vi "svx_Continuous Multitone Waveform.vi"(6 "sampling info":cluster{"Fs":dbl, "#s":dbl}={"Fs"=1000.0, "#s"=1000.0} {"Fs" format="%.2p"}, 7 "generation control":T2(ring), 8 "error in":errorcluster, 9 "delay until transition (0 samples)":i32, 10 "initial waveform state":T1 {"relative amplitudes" format="%.2p"; "frequencies" format="%.2p"; "tf" format="%.2f"; "offset" format="%.2f"; "phases" format="%.2f"; "total amplitude" format="%.2f"}, 11 "desired waveform state":T3={"frequencies"=[], "relative amplitudes"=[], "phases"=[], "total amplitude"=1.0, "offset"=0.0, "tf (ignored)"=0.0} {"relative amplitudes" format="%.2p"; "frequencies" format="%.2p"; "tf (ignored)" format="%.2f"; "phases" format="%.2f"; "offset" format="%.2p"; "total amplitude" format="%.2p"}) -> (0 "error out":errorcluster, 1 "index of transition":i32, 2 "final waveform state":T1 {"relative amplitudes" format="%.2p"; "frequencies" format="%.2p"; "tf" format="%.2f"; "offset" format="%.2f"; "phases" format="%.2f"; "total amplitude" format="%.2f"}, 3 "signal out":waveform(dbl))   [LabVIEW 2017]
uses:
  <vilib>/Analysis/NI_AALBase.lvlib
panel:
  # "You cannot change the number of tones\nand maintain continuity"
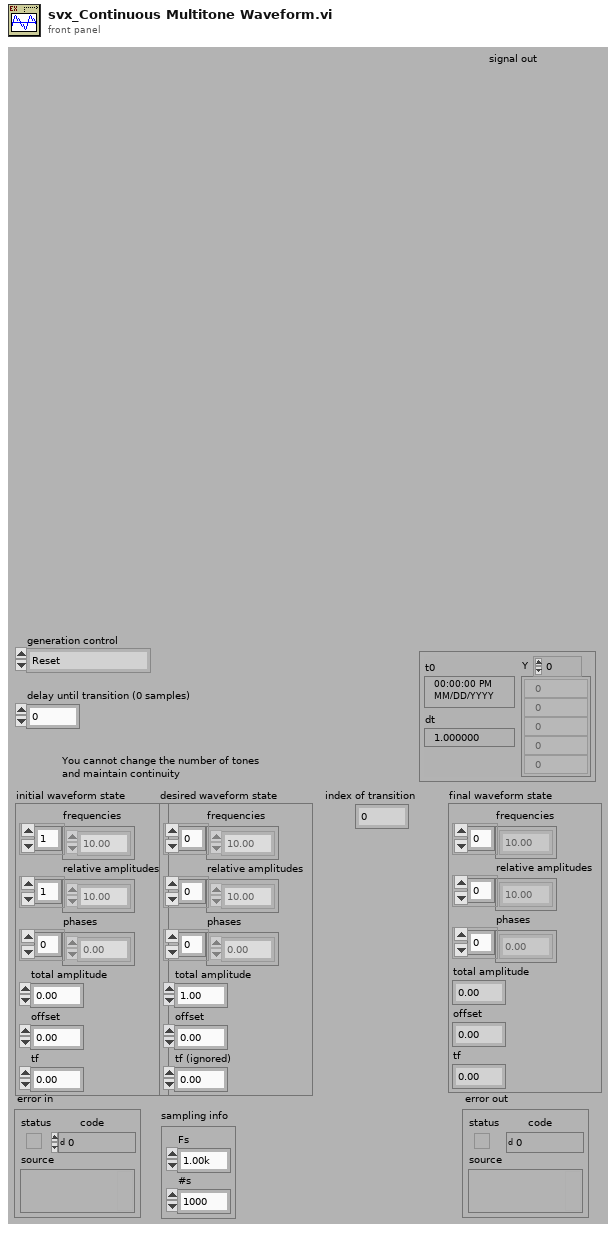
[diagram p1: front panel]
types:
  T1 = cluster{"frequencies":dbl[], "relative amplitudes":dbl[], "phases":dbl[], "total amplitude":dbl, "offset":dbl, "tf":dbl}
  T2 = enum16{"Reset", "Continue from previous", "Continue from state", "Zero from previous", "Zero from state"}
  T3 = cluster{"frequencies":dbl[], "relative amplitudes":dbl[], "phases":dbl[], "total amplitude":dbl, "offset":dbl, "tf (ignored)":dbl}
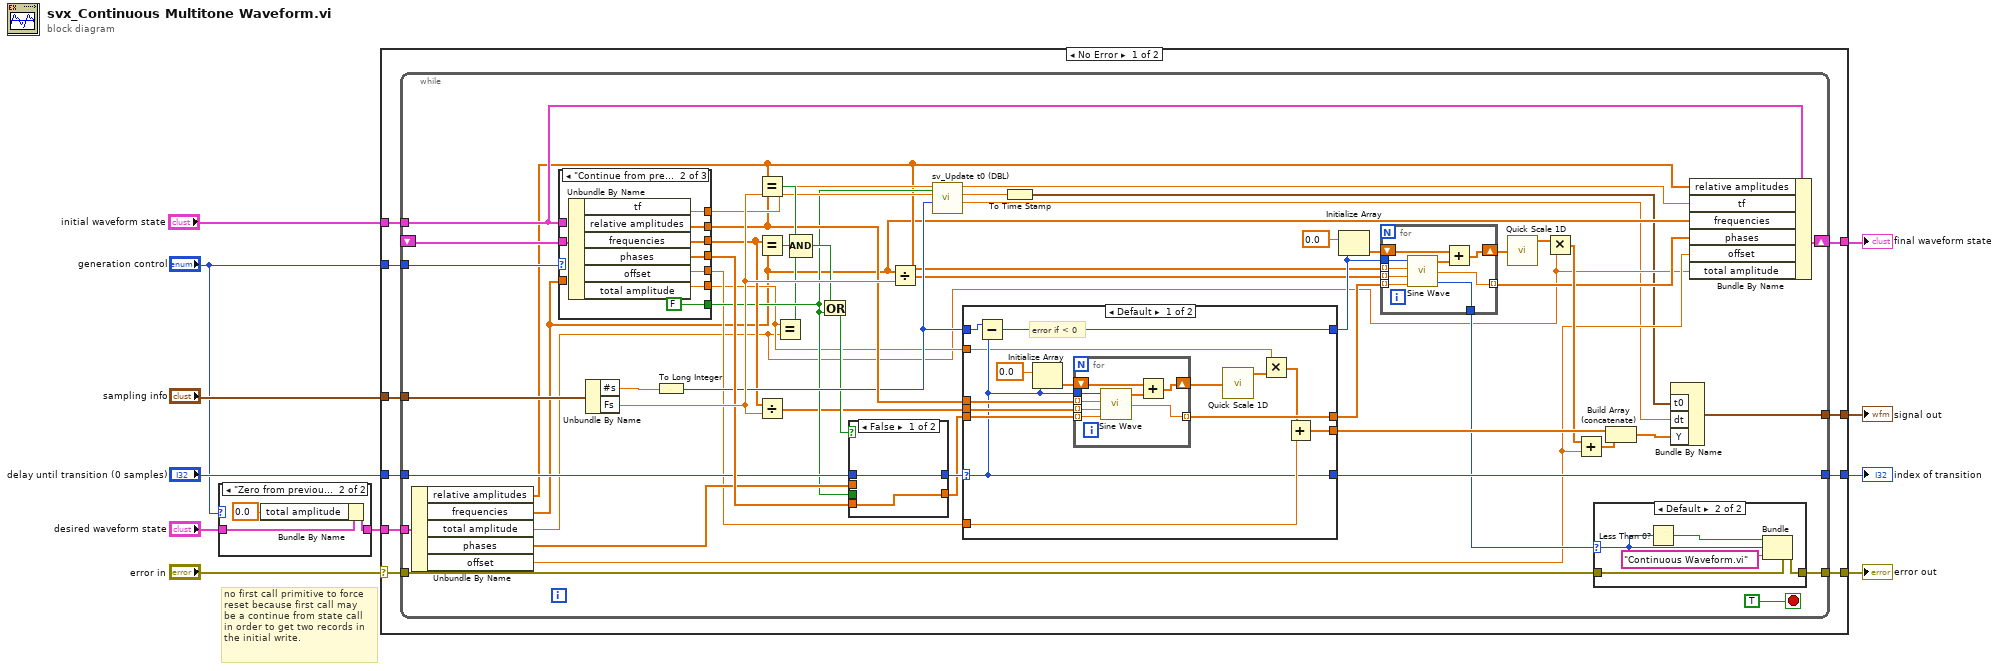
[diagram p0: block diagram]
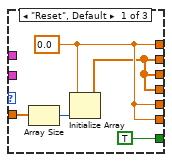
[diagram p4: hidden frame]
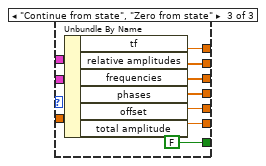
[diagram p5: hidden frame]
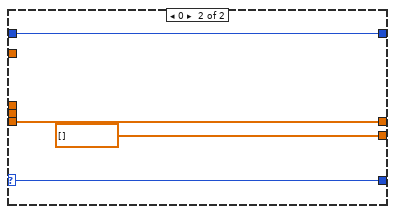
[diagram p6: hidden frame]
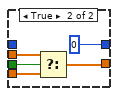
[diagram p7: hidden frame]
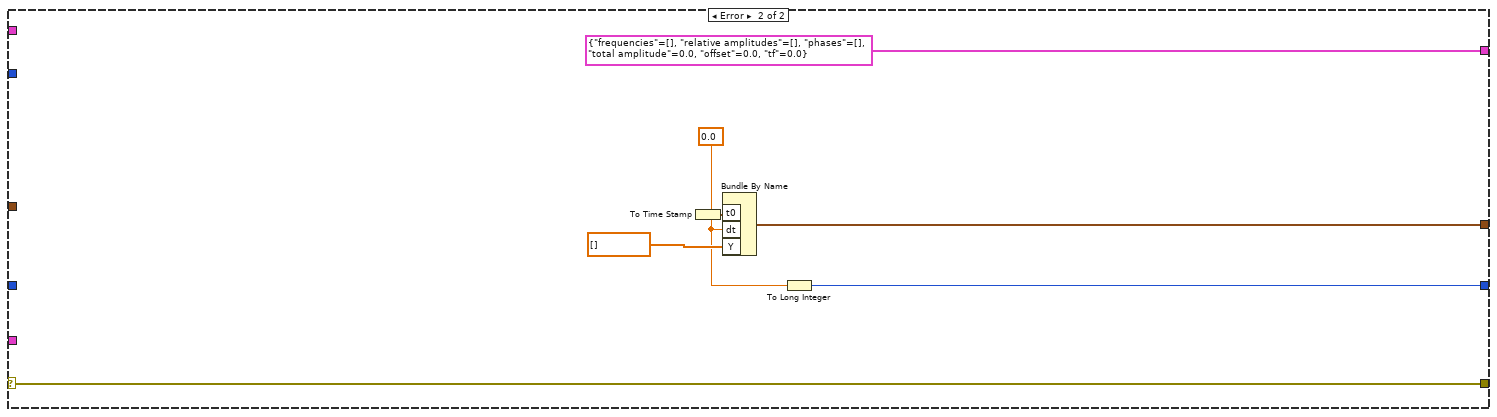
[diagram p8: hidden frame]
diagram:
  # "no first call primitive to force \nreset because first call may \nbe a continue from state call\nin order to get two records in \nthe initial write."
  n1 = case shown="\"Zero from previous\", \"Zero from state\"" "generation control" {
    tunnel: "desired waveform state" -> [w12 w14]
    tunnel: [w12 w13] -> w3
    frame Default {
    }
    frame "Zero from previous", "Zero from state" {
      n2 = Bundle By Name(cluster=w14, "total amplitude"=0.0) -> (w13:T3)
    }
  }
  n3 = case shown="No Error" "error in" {
    selector: "error in" -> [w22 w153]
    tunnel: "sampling info" -> [w25 _]
    tunnel: [w24 w153] -> w10
    tunnel: [w23 w154] -> w2
    tunnel: [w21 w150] -> w9
    tunnel: "delay until transition (0 samples)" -> [w20 _]
    tunnel: [w19 T1 {"frequencies"=[], "relative amplitudes"=[], "phases"=[], "total amplitude"=0.0, "offset"=0.0, "tf"=0.0} ("initial waveform state")] -> w7
    tunnel: "generation control" -> [w18 _]
    tunnel: w3 -> [w17 _]
    tunnel: "initial waveform state" -> [w16 _]
    frame No Error {
      n4 = while {
        tunnel: w16 -> [w52]
        tunnel: w17 -> [w60]
        tunnel: w18 -> [w67]
        shift-left: _ -> [w66]
        shift-right: [w32] -> w19
        tunnel: w20 -> [w57]
        tunnel: [w73] -> w21
        tunnel: w22 -> [w50]
        tunnel: [w75] -> w23
        tunnel: [w49] -> w24
        tunnel: w25 -> [w76]
        stop <- TRUE stop-if-true
        n5 = Unbundle By Name(w60) -> ("relative amplitudes"=w30:dbl[], "frequencies"=w29:dbl[], "total amplitude"=w28:dbl, "phases"=w59:dbl[], "offset"=w31:dbl)
        n6 = case shown="\"Continue from previous\", \"Zero from previous\"" w67 {
          tunnel: w66 -> [_ w104 _]
          tunnel: [TRUE FALSE FALSE] -> w54
          tunnel: [w94 w99 w108] -> w65
          tunnel: [w93 w103 w110] -> w64
          tunnel: [w93 w102 w112] -> w56
          tunnel: [w93 w101 w109] -> w63
          tunnel: [w94 w100 w111] -> w51
          tunnel: w52 -> [_ _ w107]
          tunnel: w29 -> [w95 _ _]
          tunnel: [w94 w98 w106] -> w38
          frame "Reset", Default {
            w94 = 0.0
            n7 = Array Size(array=w95) -> (size(s)=w96:i32)
            n8 = Initialize Array(w94, w96) -> (w93:dbl[])
          }
          frame "Continue from previous", "Zero from previous" {
            n9 = Unbundle By Name(w104) -> ("tf"=w99:dbl, "relative amplitudes"=w103:dbl[], "frequencies"=w102:dbl[], "phases"=w101:dbl[], "offset"=w100:dbl, "total amplitude"=w98:dbl)
          }
          frame "Continue from state", "Zero from state" {
            n10 = Unbundle By Name(w107) -> ("tf"=w108:dbl, "relative amplitudes"=w110:dbl[], "frequencies"=w112:dbl[], "phases"=w109:dbl[], "offset"=w111:dbl, "total amplitude"=w106:dbl)
          }
        }
        n11 = Unbundle By Name(w76) -> ("#s"=w58:dbl, "Fs"=w71:dbl)
        n12 = To Long Integer(number=w58) -> (32bit integer=w61:i32)
        n13 = Equal?(x=w30, y=w64) -> (x = y?=w74:bool)
        n14 = Equal?(x=w56, y=w29) -> (x = y?=w41:bool)
        n15 = Divide(x=w56, y=w71) -> (x/y=w48:dbl[])
        n16 = Equal?(x=w38, y=w28) -> (x = y?=w40:bool)
        n17 = Compound Arithmetic op=AND(w74, w41, w40) -> (w55:bool)
        n18 = Or(x=w55, y=w54) -> (x .or. y?=w53:bool)
        n19 = case shown="False" w53 {
          tunnel: [w142 w143] -> w34
          tunnel: w63 -> [w142 w144]
          tunnel: w57 -> [w141 _]
          tunnel: w59 -> [_ w145]
          tunnel: [w141 0] -> w47
          tunnel: w54 -> [_ w146]
          frame False {
          }
          frame True {
            n20 = Select(t=w145, s=w146, f=w144) -> (s? t:f=w143:dbl[])
          }
        }
        n21 = Divide(x=w29, y=w71) -> (x/y=w43:dbl[])
        n22 = call <vilib>:"sv_Update t0 (DBL).vi"("Reset Generation"=w54, "samples"=w61, "sample rate (S/s)"=w71, "tf previous"=w65) -> ("dt"=w26:dbl, "t0"=w62:dbl, "tf new"=w68:dbl)  [unwired: 5 in]
        n23 = case shown="Default" w47 {
          selector: w47 -> [w118 w137]
          tunnel: [w124 w138] -> w39
          tunnel: w61 -> [w125 w139]
          tunnel: w64 -> [w128 _]
          tunnel: [w118 w137] -> w73
          tunnel: [w126 dbl[] [] ("Sine Wave")] -> w72
          tunnel: [w127 w139] -> w46
          tunnel: w48 -> [w122 _]
          tunnel: w51 -> [w123 _]
          tunnel: w34 -> [w121 w138]
          tunnel: w38 -> [w115 _]
          frame Default {
            # "error if < 0"
            n24 = Subtract(x=w125, y=w118) -> (x-y=w127:i32)
            n25 = Initialize Array(0.0 ("element"), w118) -> (w119:dbl[])
            n26 = for {
              tunnel: w128 -> [w136] mode=indexing
              tunnel: w122 -> [w135] mode=indexing
              tunnel: w121 -> [w134] mode=indexing
              tunnel: w118 -> [w133]
              tunnel: [w132] -> w124 mode=indexing
              shift-right: [w129] -> w117
              shift-left: w119 -> [w131]
              n27 = call <vilib>:"Sine Wave.vi"("samples"=w133, "amplitude"=w136, "frequency"=w135, "phase in"=w134) -> ("sine wave"=w130:dbl[], "phase out"=w132:dbl)  [unwired: 1 in, 1 out]
              n28 = Add(x=w131, y=w130) -> (x+y=w129:dbl[])
            }
            n29 = call <vilib>:"Quick Scale 1D.vi"("X"=w117) -> ("Y[i]=X[i]/Max|X|"=w116:dbl[])  [unwired: 2 out]
            n30 = Multiply(x=w115, y=w116) -> (x*y=w114:dbl[])
            n31 = Add(x=w114, y=w123) -> (x+y=w126:dbl[])
          }
          frame 0 {
          }
        }
        n32 = To Time Stamp(1:w62) -> (0:w27:timestamp)
        n33 = Initialize Array(0.0 ("element"), w46) -> (w45:dbl[])
        n34 = for {
          tunnel: w30 -> [w86] mode=indexing
          tunnel: w43 -> [w85] mode=indexing
          tunnel: w39 -> [w84] mode=indexing
          tunnel: w46 -> [w83]
          tunnel: [w82] -> w33 mode=indexing
          shift-right: [w79] -> w37
          shift-left: w45 -> [w81]
          tunnel: [w78] -> w42
          n35 = call <vilib>:"Sine Wave.vi"("samples"=w83, "amplitude"=w86, "frequency"=w85, "phase in"=w84) -> ("sine wave"=w80:dbl[], "phase out"=w82:dbl, "error"=w78:i32)  [unwired: 1 in]
          n36 = Add(x=w81, y=w80) -> (x+y=w79:dbl[])
        }
        n37 = call <vilib>:"Quick Scale 1D.vi"("X"=w37) -> ("Y[i]=X[i]/Max|X|"=w35:dbl[])  [unwired: 2 out]
        n38 = Multiply(x=w35, y=w28) -> (x*y=w36:dbl[])
        n39 = Add(x=w36, y=w31) -> (x+y=w70:dbl[])
        n40 = case shown="Default" w42 {
          selector: w42 -> [_ w91]
          tunnel: w50 -> [w87 w92]
          tunnel: [w87 w88] -> w49
          frame 0 {
          }
          frame Default {
            n41 = Less Than 0?(x=w91) -> (x < 0?=w90:bool)
            n42 = Bundle(cluster=w92, "status"=w90, "code"=w91, "source"="Continuous Waveform.vi" ("subVI Name")) -> (w88:errorcluster)
          }
        }
        n43 = Build Array (concatenate)(w72, w70) -> (w69:dbl[])
        n44 = Bundle By Name("t0"=w27, "dt"=w26, "Y"=w69) -> (w75:waveform(dbl))  [unwired: 1 in]
        n45 = Bundle By Name(cluster=w52, "relative amplitudes"=w30, "tf"=w68, "frequencies"=w29, "phases"=w33, "offset"=w31, "total amplitude"=w28) -> (w32:T1)
      }
    }
    frame Error {
      w151 = 0.0 ("t0")
      n46 = To Time Stamp(1:w151) -> (0:w148:timestamp)
      n47 = Bundle By Name("t0"=w148, "dt"=w151, "Y"=dbl[] []) -> (w154:waveform(dbl))  [unwired: 1 in]
      n48 = To Long Integer(number=w151) -> (32bit integer=w150:i32)
    }
  }
  "error out" <- w10
  "signal out" <- w2
  "index of transition" <- w9
  "final waveform state" <- w7
